vi "SeCrTs-DI_Read.vi"(8 "error in (no error)":errorcluster, 9 "number of samples per channel":i32, 10 "DI_Task":refnum<k21>, 11 "Data FIFO Ref":T1) -> (0 "error out":errorcluster, 2 "task out":refnum<k21>)   [LabVIEW 2022 SP3]
uses:
  RT Controls/SeCrTs-Data FIFO.ctl
  <vilib>/Platform/TimedLoop/XDataNode/timing_clust.ctl
  <vilib>/Platform/TimedLoop/XDataNode/nitl_modes.ctl
  <vilib>/Platform/TimedLoop/XDataNode/wakeup.ctl
  RT Controls/SeCrTs-FGV Read write.ctl
  <vilib>/DAQmx/read.llb/DAQmx Read (Digital 1D Wfm NChan NSamp).vi
  <vilib>/DAQmx/miscellaneous.llb/DAQmx Fill In Error Info.vi
  <vilib>/Waveform/DTblOps.llb/DTbl Digital to Boolean Array.vi
  <vilib>/platform/TimedLoop/XDataNode/XDataNode.xnode
  <vilib>/Platform/TimedLoop/XDataNode/XDNodeRunTimeDep.lvlib
panel:
  out "overflow?":bool
  out "x-y":u32
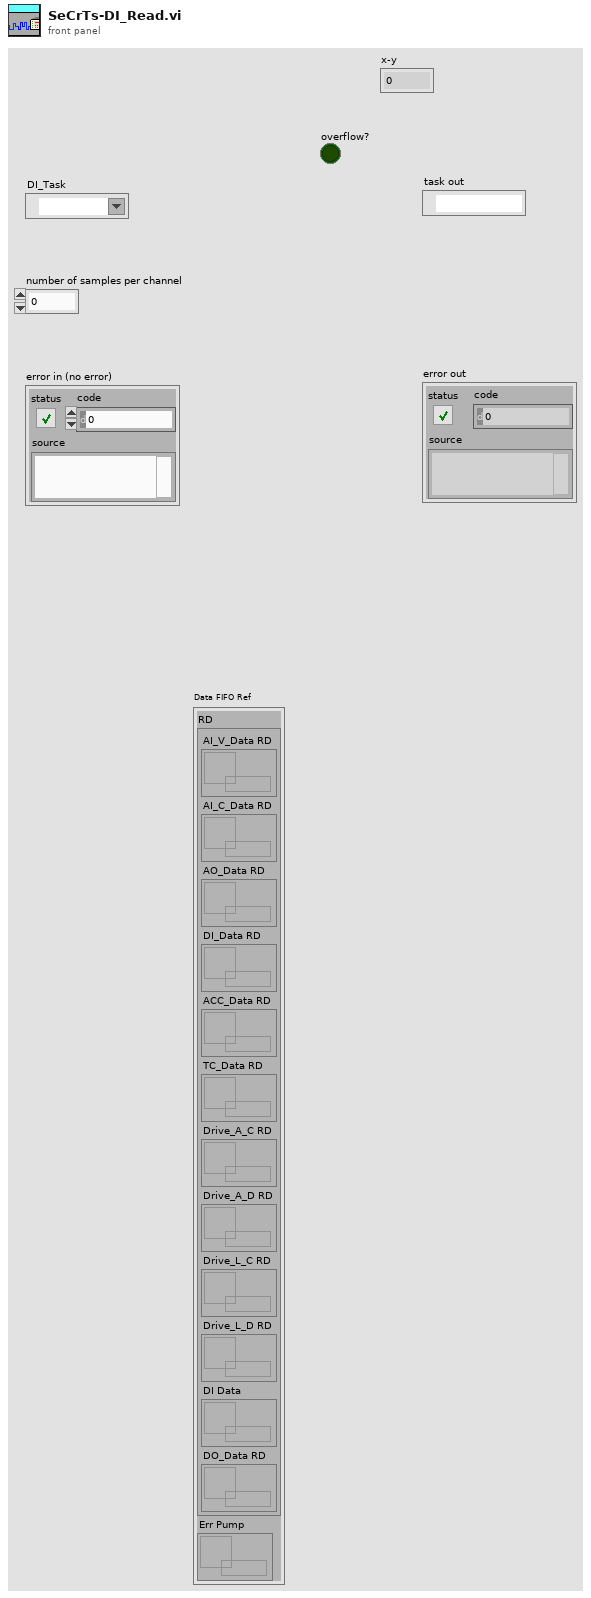
[diagram p1: front panel]
types:
  T1 = typedef "SeCrTs-Data FIFO.ctl" = cluster{"RD":cluster{"AI_V_Data RD":refnum<queue>, "AI_C_Data RD":refnum<queue>, "AO_Data RD":refnum<queue>, "DI_Data RD":refnum<queue>, "ACC_Data RD":refnum<queue>, "TC_Data RD":refnum<queue>, "Drive_A_C RD":refnum<queue>, "Drive_A_D RD":refnum<queue>, "Drive_L_C RD":refnum<queue>, "Drive_L_D RD":refnum<queue>, "DI Data":refnum<queue>, "DO_Data RD":refnum<queue>}, "Err Pump":refnum<queue>}
  T2 = cluster{"AO config":cluster{"Channel_Name":string, "Channel_Number":string, "Default_Value":dbl, "Units":string}[], "AI config":cluster{"Channel_Name":string, "Channel_Number":string, "Pre_Scale_min":dbl, "Pre_Scale_max":dbl, "Sensor_min":dbl, "Sensor_max":dbl, "Units":string}[], "DI config":cluster{"Channel_Name":string, "Channel_Number":string, "Default_Value":bool, "DI invert?":bool}[], "DO config":cluster{"Channel_Name":string, "Channel_Number":string, "Default_Value":bool, "DO invert?":bool}[], "TC config":cluster{"Channel_Name":string, "Channel_Number":string, "Pre_Scale_min":dbl, "Pre_Scale_max":dbl, "units":i32, "thermocouple type":i32}[], "ACC config":cluster{"Channel_Name":string, "Channel_Number":string, "Pre_Scale_min":dbl, "Pre_Scale_max":dbl, "Terminal configuration":i32, "Sensitivity":dbl, "Sensitivity units":i32}[], "SG config":cluster{"Channel_Name":string, "Channel_Number":string, "Pre_Scale_min":dbl, "Pre_Scale_max":dbl}[], "Strain Gauge Settings":cluster{"poisson ratio":dbl, "nominal gage resistance":dbl, "gage factor":dbl}, "Bridge Settings":cluster{"voltage excitation value":dbl, "voltage excitation source":i32, "initial bridge voltage":dbl, "lead wire resistance":dbl, "strain configuration":i32}, "Sample Rate":cluster{"AI Sample Rate":dbl[], "AO Sample Rate":dbl[], "DI Sample Rate":dbl[], "TC Sample Rate":dbl[], "DO Sample Rate":dbl[], "SG Sample Rate":dbl[], "ACC Sample Rate":dbl[]}}
  T3 = cluster{"Channel_Name":string, "Channel_Number":string, "Default_Value":bool, "DI invert?":bool}[]
  T4 = typedef "XDNodeRunTimeDep.lvlib/timing_clust.ctl" = cluster{"Expected End [f-1]":u64, "Actual End [f-1]":u64, "Finished Late? [f-1]":bool, "Expected End [i-1]":u64, "Actual End [i-1]":u64, "Finished Late? [i-1]":bool, "Expected Start [i]":u64, "Actual Start [i]":u64, "Expected Start [f]":u64, "Actual Start [f]":u64, "Source Name":string, "Structure Name":string, "Period":i64, "Deadline":i64, "Offset":i64, "Start":i64, "Priority":i32, "Timeout":i32, "Mode":T5, "Wakeup Reason":T6, "Error":errorcluster, "Source Type":string, "Secondary Source Type":string, "Global End Time":u64, "Global Start Time":u64, "Frame Duration":u64, "Iteration Duration":u64, "Assigned CPU":i32, "I/O Scan Engine Mode":u32}
  T5 = typedef "XDNodeRunTimeDep.lvlib/nitl_modes.ctl" = enum32{"No Change", "Process missed periods, maintain original phase", "Discard missed periods, maintain original phase", "Process missed periods, ignore original phase", "Discard missed periods, ignore original phase"}
  T6 = typedef "XDNodeRunTimeDep.lvlib/wakeup.ctl" = enum32{"Normal", "Aborted", "Asynchronous wakeup", "Timing source error", "Timed loop error", "Timeout"}
  T7 = enum16{"AI C", "AI V", "AO", "DI", "DO", "TC", "ACC", "RT PMP", "DR A"}
  T8 = typedef "SeCrTs-FGV Read write.ctl" = enum16{"Write", "Read"}
  T9 = enum16{"Init", "Read 'All'", "Read 'n'", "Read '1'", "Write '1'", "Write 'n'", "Write 'All'"}
  T10 = cluster{"Start DAQ":bool, "Stop DAQ":bool, "RT Stop":bool, "RT Exit":bool, "Start Seq":bool}
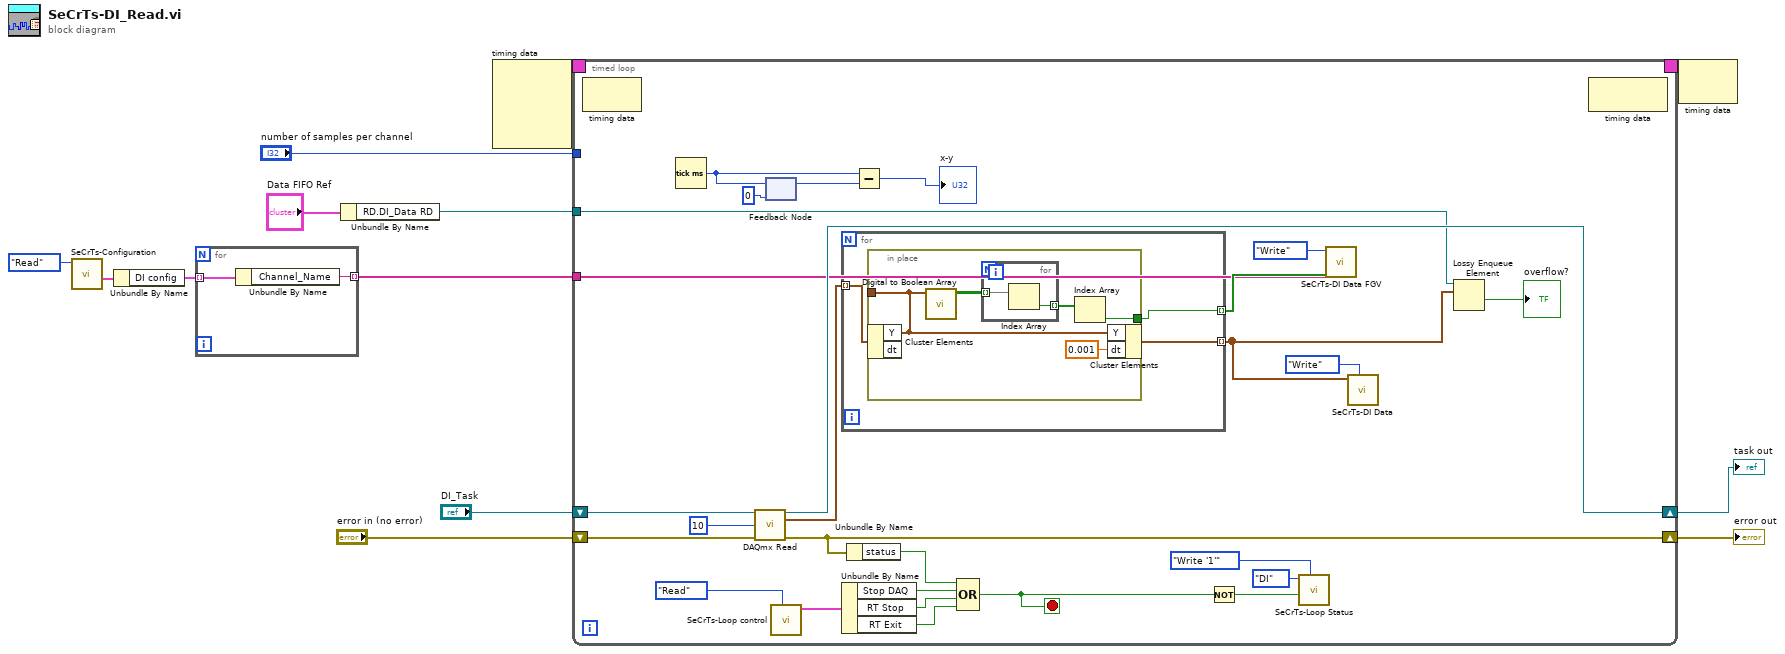
[diagram p0: block diagram]
diagram:
  n1 = call "SeCrTs-Configuration.vi"("Enum"=enum16{"Write", "Read"}."Read") -> ("Config out"=w7:T2)  [unwired: 10 in]
  n2 = Unbundle By Name(w7) -> ("DI config"=w6:T3)
  n3 = for {
    tunnel: w6 -> [w15] mode=indexing
    tunnel: [w14] -> w5 mode=indexing
    n4 = Unbundle By Name(w15) -> ("Channel_Name"=w14:string)
  }
  n5 = Unbundle By Name("Data FIFO Ref") -> ("RD.DI_Data RD"=w3:refnum<queue>)
  n6 = node-c288() -> (w2:T4)  [unwired: 4 in]
  n7 = timed-loop {
    tunnel: "number of samples per channel" -> [_]
    tunnel: w3 -> [w21]
    shift-right: [w26] -> w10
    shift-left: "DI_Task" -> [w41]
    shift-right: [w19] -> w9
    shift-left: "error in (no error)" -> [w40]
    tunnel: w5 -> [w24]
    timing: w2 -> [_]
    timing-out: [_] -> w1
    stop <- w42 stop-if-true
    n8 = node-c288() -> ()  [unwired: 1 in, 1 out]
    n9 = Tick Count (ms)() -> (millisecond timer value=w31:u32)
    n10 = call-poly <vilib>:"DAQmx Read.vi"("task/channels in"=w41, "number of samples per channel"=10, "error in"=w40) -> ("task out"=w26:refnum<k21>, "data"=w18:digitalwaveform[], "error out"=w19:errorcluster)  [unwired: 10 in]
    n11 = feedback-in #1(w31) -> ()
    n12 = feedback #1(u32 0 ("millisecond timer value")) -> (w30:u32)
    n13 = call "SeCrTs-Loop control.vi"("Action"=enum16{"Init", "Write", "Read"}."Read") -> ("Loop Control out"=w34:T10)  [unwired: 9 in, 1 out]
    n14 = for {
      tunnel: w18 -> [w46] mode=indexing
      tunnel: [w47] -> w25 mode=indexing
      tunnel: [w45] -> w17 mode=indexing
      n15 = in-place {
        in-place-border: [w52] -> w47
        in-place-border: [w48] -> _
        n16 = in-place-cluster #2(w46) -> ("Y"=w48:digitaldata)  [unwired: 1 out]
        n17 = call-poly <vilib>:"Digital to Boolean Array.vi"("digital data"=w48) -> ("boolean array"=w50:bool[][])  [unwired: 9 in, 1 out]
        n18 = for {
          tunnel: w50 -> [w54] mode=indexing
          tunnel: [w53] -> w51 mode=indexing
          n19 = Index Array(array=w54) -> (element=w53:bool)  [unwired: 1 in]
        }
        n20 = Index Array(array=w51) -> (element=w52:bool)  [unwired: 1 in]
        n21 = in-place-cluster #2("Y"=w48, "dt"=0.001) -> (w45:digitalwaveform)
      }
    }
    n22 = Unbundle By Name(w34) -> ("Stop DAQ"=w38:bool, "RT Stop"=w37:bool, "RT Exit"=w36:bool)
    n23 = Unbundle By Name(w19) -> ("status"=w39:bool)
    n24 = Subtract(x=w31, y=w30) -> (x-y=→"x-y":u32)
    n25 = Compound Arithmetic op=OR(w39, w38, w37, w36) -> (w42:bool)
    n26 = Not(x=w42) -> (.not. x?=w32:bool)
    n27 = call "SeCrTs-Loop Status.vi"("Option"=T9."Write '1'", "Status"=w32, "Loop"=T7."DI") -> ()  [unwired: 6 in, 3 out]
    n28 = call "SeCrTs-DI Data FGV.vi"("DI Y LP"=w25, "DI Signal List LP"=w24, "Write/Read"=SeCrTs-FGV_Read_write."Write") -> ()  [unwired: 6 in, 3 out]
    n29 = call "SeCrTs-DI Data.vi"("Enum"=enum16{"Write", "Read"}."Write", "In_DI data"=w17) -> ()  [unwired: 9 in, 1 out]
    n30 = Lossy Enqueue Element(queue=w21, element=w17) -> (overflow?=→"overflow?":bool)  [unwired: 1 in, 3 out]
    n31 = node-c288() -> ()  [unwired: 1 in, 1 out]
  }
  "task out" <- w10
  "error out" <- w9
  n32 = node-c288(w1) -> ()  [unwired: 1 out]
